vi "Non_Displayable_var.vi"(1 "Attribute Name Array":string[](array[string])) -> (0 "Output Attribute Array":string[][](array[string]))   [LabVIEW 2020]
panel:
  in  "NA":string="Non Displayable"
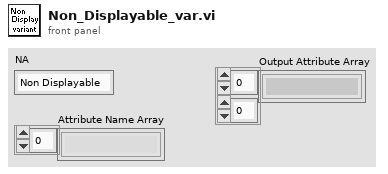
[diagram p1: front panel]
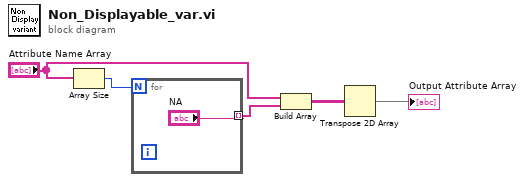
[diagram p0: block diagram]
diagram:
  n1 = Array Size(array="Attribute Name Array") -> (size(s)=w1:i32)
  n2 = for {
    N: w1 -> [_]
    tunnel: ["NA"] -> w2 mode=indexing
  }
  n3 = Build Array("Attribute Name Array", w2) -> (w3:string[][])
  n4 = Transpose 2D Array(2D array=w3) -> (transposed array=→"Output Attribute Array":string[][])
